vi "SP Append Filter Bandwidth Limit Waveform.vi"(4 "Limit Format":T2, 6 "Measured Parameter":T4={"Stimulus Port"=1, "Response Port"=1} {"Stimulus Port" min=1 step=1; "Response Port" min=1 step=1}, 7 "Attribute Name (NI_ChannelName)":string="NI_ChannelName", 8 "error in (no error)":errorcluster, 9 "Filter Type":T1=enum."Bandpass", 10 "Results":T3, 11 "Waveforms in":waveform(dbl)[](array[waveform])) -> (0 "error out":errorcluster, 3 "Waveforms out":waveform(dbl)[](array[waveform]))   [LabVIEW 2011]
uses:
  TypeDefs/SP Parameter.ctl
  TypeDefs/SP Format.ctl
  TypeDefs/SP Filter Type.ctl
  Channel Test Status Enumeration.ctl
  TypeDefs/SP Channel Type.ctl
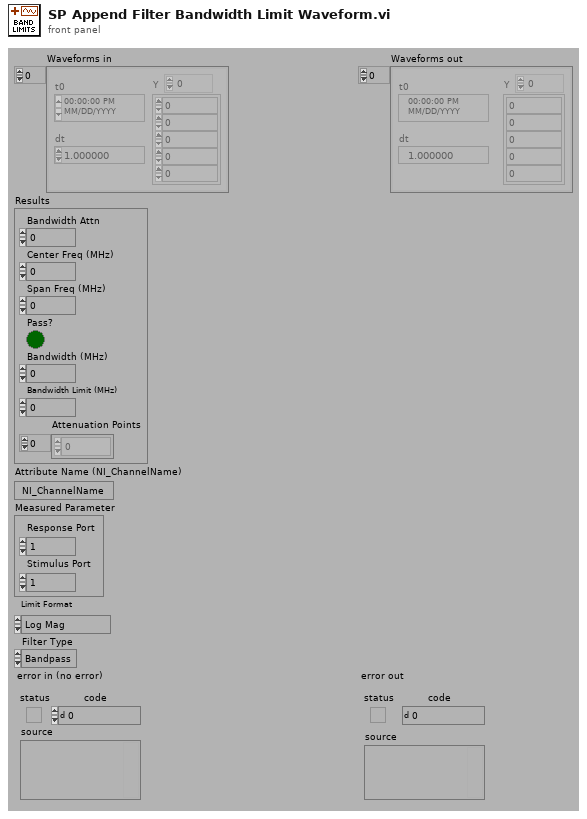
[diagram p1: front panel]
types:
  T1 = typedef "SP Filter Type.ctl" = enum16{"Lowpass", "Highpass", "Bandpass", "Bandstop"}
  T2 = typedef "SP Format.ctl" = enum16{"Log Mag", "Lin Mag", "SWR", "Phase", "Expanded Phase", "Delay", "Insertion Loss", "Isolation", "Return Loss"}
  T3 = cluster{"Bandwidth Attn":dbl, "Center Freq (MHz)":dbl, "Span Freq (MHz)":dbl, "Pass?":bool, "Bandwidth (MHz)":dbl, "Bandwidth Limit (MHz)":dbl, "Attenuation Points":dbl[]}
  T4 = typedef "SP Parameter.ctl" = cluster{"Stimulus Port":i8, "Response Port":i8}
  T5 = typedef "SP Channel Type.ctl" = enum16{"Frequency", "Data", "Limit", "Adapter", "Memory", "Value", "Value Limit"}
  T6 = typedef "Channel Test Status Enumeration.ctl" = enum16{"Fail", "Pass", "Abort", "Error", "Done", "Pass by Sample", "Fail by Sample", "Pass Override", "Fail Override", "Not Tested"}
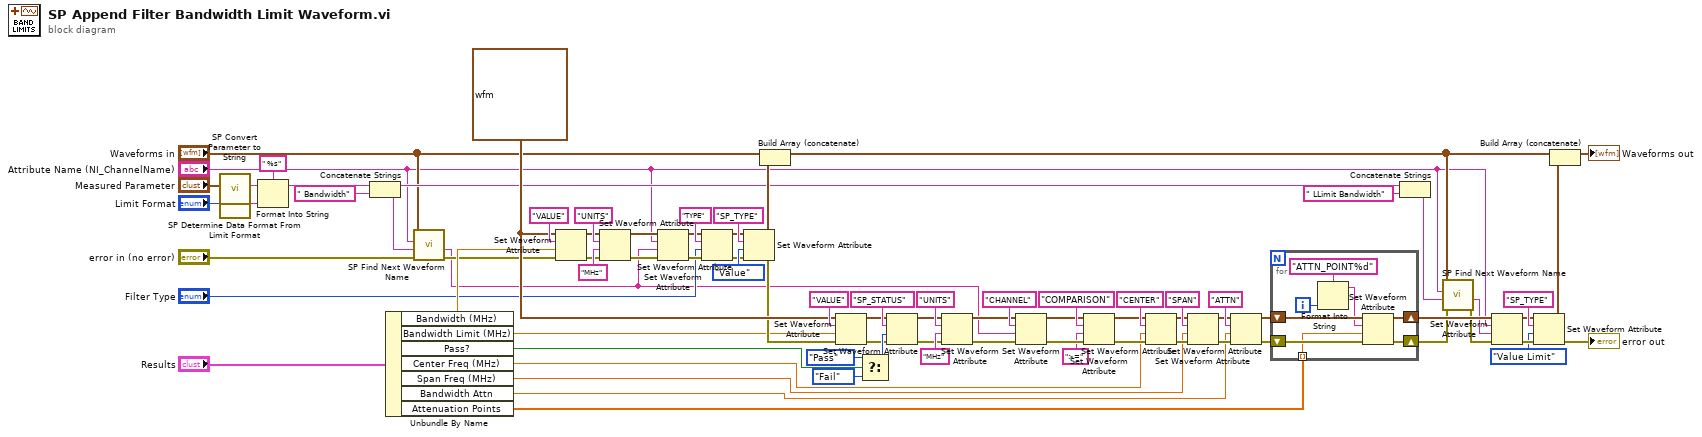
[diagram p0: block diagram]
diagram:
  w51 = waveform(dbl) {"t0"=timestamp(0 s since 1904-01-01), "dt"=1.0, "Y"=[]} ("waveform")
  n1 = call "SP Convert Parameter to String.vi"("Parameter"="Measured Parameter") -> ("Parameter String"=w41:string)  [unwired: 10 out]
  n2 = call "SP Determine Data Format From Limit Format.vi"("Limit Format"="Limit Format") -> ("Format String"=w38:string)
  n3 = Format Into String(format string=" %s", initial string=w41, w38) -> (resulting string=w40:string)  [unwired: 1 in, 1 out]
  n4 = Concatenate Strings(w40, " Bandwidth") -> (w8:string)
  n5 = Unbundle By Name("Results") -> ("Bandwidth (MHz)"=w36:dbl, "Bandwidth Limit (MHz)"=w35:dbl, "Pass?"=w34:bool, "Center Freq (MHz)"=w22:dbl, "Span Freq (MHz)"=w23:dbl, "Bandwidth Attn"=w24:dbl, "Attenuation Points"=w12:dbl[])
  n6 = call "SP Find Next Waveform Name.vi"("error in (no error)"="error in (no error)", "Prospective Base Name"=w8, "Attribute Name (NI_ChannelName)"="Attribute Name (NI_ChannelName)", "Waveforms in"="Waveforms in") -> ("error out"=w10:errorcluster, "Channel Name"=w7:string)  [unwired: 6 in]
  n7 = Set Waveform Attribute(4:w10, 5:w36, 6:"VALUE", 7:w51) -> (0:w57:errorcluster, 3:w60:waveform(dbl))  [unwired: 1 out]
  n8 = Set Waveform Attribute(4:w57, 5:"MHz", 6:"UNITS", 7:w60) -> (0:w58:errorcluster, 3:w59:waveform(dbl))  [unwired: 1 out]
  n9 = Set Waveform Attribute(4:w58, 5:w7, 6:"Attribute Name (NI_ChannelName)", 7:w59) -> (0:w19:errorcluster, 3:w20:waveform(dbl))  [unwired: 1 out]
  n10 = Set Waveform Attribute(4:w19, 5:"Filter Type", 6:"TYPE", 7:w20) -> (0:w18:errorcluster, 3:w17:waveform(dbl))  [unwired: 1 out]
  n11 = Set Waveform Attribute(4:w18, 5:SP_Channel_Type."Value" ("Channel Type"), 6:"SP_TYPE", 7:w17) -> (0:w50:errorcluster, 3:w68:waveform(dbl))  [unwired: 1 out]
  n12 = Build Array (concatenate)("Waveforms in", w68) -> (w4:waveform(dbl)[])
  n13 = Set Waveform Attribute(4:w50, 5:w35, 6:"VALUE", 7:w51) -> (0:w49:errorcluster, 3:w48:waveform(dbl))  [unwired: 1 out]
  n14 = Select(t=Channel_Test_Status_Enumeration."Pass" ("Channel Status Enumeration"), s=w34, f=Channel_Test_Status_Enumeration."Fail" ("Channel Status Enumeration")) -> (s? t:f=w76:T6)
  n15 = Set Waveform Attribute(4:w49, 5:w76, 6:"SP_STATUS", 7:w48) -> (0:w61:errorcluster, 3:w62:waveform(dbl))  [unwired: 1 out]
  n16 = Set Waveform Attribute(4:w61, 5:"MHz", 6:"UNITS", 7:w62) -> (0:w55:errorcluster, 3:w54:waveform(dbl))  [unwired: 1 out]
  n17 = Set Waveform Attribute(4:w55, 5:w7, 6:"CHANNEL", 7:w54) -> (0:w45:errorcluster, 3:w46:waveform(dbl))  [unwired: 1 out]
  n18 = Set Waveform Attribute(4:w45, 5:">=", 6:"COMPARISON", 7:w46) -> (0:w30:errorcluster, 3:w25:waveform(dbl))  [unwired: 1 out]
  n19 = Set Waveform Attribute(4:w30, 5:w22, 6:"CENTER", 7:w25) -> (0:w29:errorcluster, 3:w26:waveform(dbl))  [unwired: 1 out]
  n20 = Set Waveform Attribute(4:w29, 5:w23, 6:"SPAN", 7:w26) -> (0:w28:errorcluster, 3:w27:waveform(dbl))  [unwired: 1 out]
  n21 = Set Waveform Attribute(4:w28, 5:w24, 6:"ATTN", 7:w27) -> (0:w14:errorcluster, 3:w15:waveform(dbl))  [unwired: 1 out]
  n22 = for {
    shift-right: [w86] -> w13
    shift-left: w15 -> [w85]
    shift-right: [w87] -> w6
    shift-left: w14 -> [w88]
    tunnel: w12 -> [w83] mode=indexing
    i -> [w89]
    n23 = Format Into String(format string="ATTN_POINT%d", w89) -> (resulting string=w84:string)  [unwired: 2 in, 1 out]
    n24 = Set Waveform Attribute(4:w88, 5:w83, 6:w84, 7:w85) -> (0:w87:errorcluster, 3:w86:waveform(dbl))  [unwired: 1 out]
  }
  n25 = Concatenate Strings(w40, " LLimit Bandwidth") -> (w2:string)
  n26 = call "SP Find Next Waveform Name.vi"("error in (no error)"=w6, "Prospective Base Name"=w2, "Attribute Name (NI_ChannelName)"="Attribute Name (NI_ChannelName)", "Waveforms in"=w4) -> ("error out"=w5:errorcluster, "Channel Name"=w1:string)  [unwired: 6 in]
  n27 = Set Waveform Attribute(4:w5, 5:w1, 6:"Attribute Name (NI_ChannelName)", 7:w13) -> (0:w73:errorcluster, 3:w74:waveform(dbl))  [unwired: 1 out]
  n28 = Set Waveform Attribute(4:w73, 5:SP_Channel_Type."Value Limit" ("Channel Type"), 6:"SP_TYPE", 7:w74) -> (0:→"error out":errorcluster, 3:w72:waveform(dbl))  [unwired: 1 out]
  n29 = Build Array (concatenate)(w4, w72) -> (→"Waveforms out":waveform(dbl)[])
